vi "Initial Droplet Charge.vi"(9 "Droplet Size":dbl, 10 "Flow Rate":dbl, 11 "Current":dbl) -> (3 "Initial Droplet Charge":dbl)   [LabVIEW 2020]
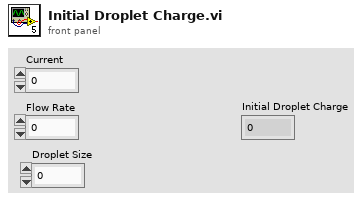
[diagram p1: front panel]
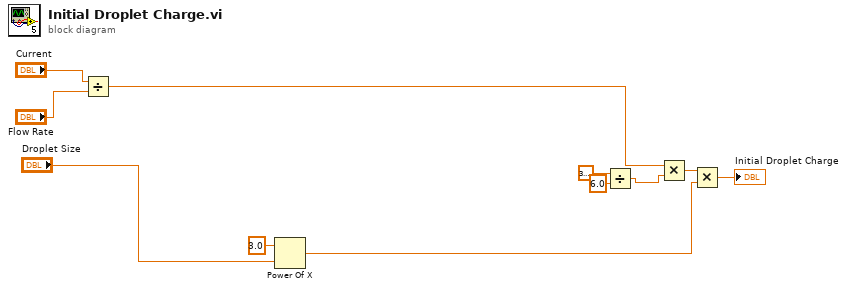
[diagram p0: block diagram]
diagram:
  n1 = Divide(x="Current", y="Flow Rate") -> (x/y=w7:dbl)
  n2 = Power Of X(1:"Droplet Size", 2:3.0 ("y")) -> (0:w2:dbl)
  n3 = Divide(x=3.141592653589793, y=6.0) -> (x/y=w6:dbl)
  n4 = Multiply(x=w7, y=w6) -> (x*y=w3:dbl)
  n5 = Multiply(x=w3, y=w2) -> (x*y=→"Initial Droplet Charge":dbl)
